vi "dragNode.vi"(8 "error in (no error)":errorcluster, 10 "Node Path":string, 11 "xceRootNode in":refnum<class "xceRootNode.lvclass">) -> (0 "error out":errorcluster, 3 "xceRootNode out":refnum<class "xceRootNode.lvclass">)   [LabVIEW 2013, in "xceRootNode.lvclass"]
doc: "Used in a drag/drop operation, when the user has detrmined which tree tag in a tree control they would like to drag."
uses:
  xceRootNode.lvclass
  xceDataNode/xceDataNode.lvclass
  xceRootNode.lvclass/xceRootNode.ctl
  xceNode/xceNode.lvclass
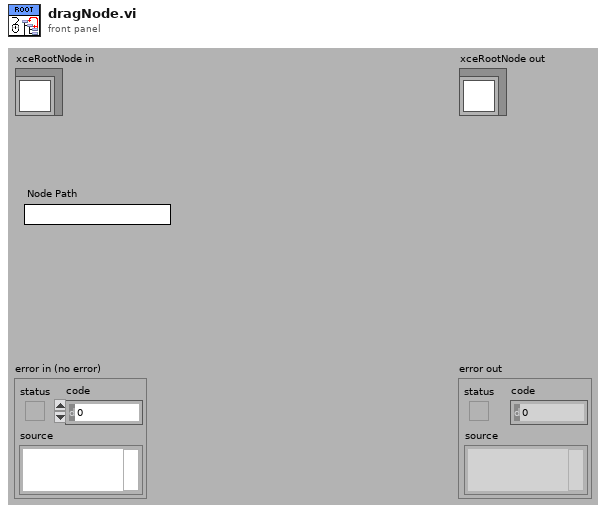
[diagram p1: front panel]
types:
  T1 = cluster{"data name":string, "drag data":variant}[]
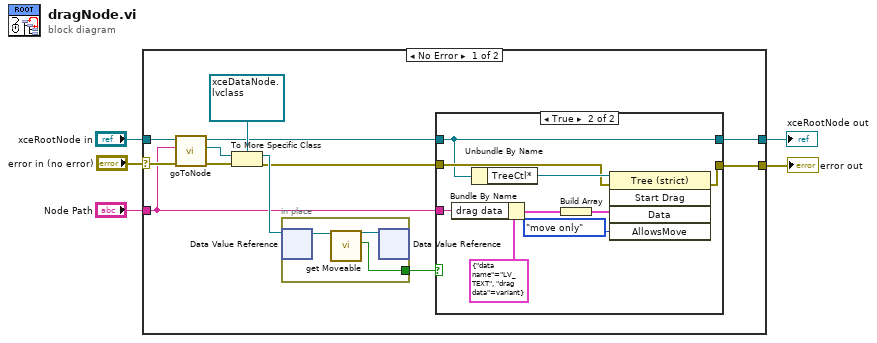
[diagram p0: block diagram]
diagram:
  n1 = case shown="No Error" "error in (no error)" {
    selector: "error in (no error)" -> [w14 w33]
    tunnel: [w8 w33] -> w4
    tunnel: [w6 w32] -> w2
    tunnel: "xceRootNode in" -> [w17 w32]
    tunnel: "Node Path" -> [w10 _]
    frame No Error {
      n2 = call "goToNode.vi"("error in (no error)"=w14, "Node Path"=w10, "xceNode in"=w17) -> ("error out"=w15:errorcluster, "goToNode* out"=w16:refnum<data-value>, "xceNode out"=w11:refnum<class "xceRootNode.lvclass">)  [unwired: 6 in]
      n3 = To More Specific Class(target class=refnum<data-value> refnum ("data value reference"), reference=w16, error in=w15) -> (specific class reference=w12:refnum<data-value>, error out=w9:errorcluster)
      n4 = in-place {
        in-place-border: [w29] -> w7
        n5 = in-place-dvr #1(w12) -> (w31:refnum<class "xceDataNode.lvclass">)  [unwired: 1 out]
        n6 = call "get Moveable.vi"("xceDataNode in"=w31) -> ("Moveable"=w29:bool, "xceDataNode out"=w30:refnum<class "xceDataNode.lvclass">)  [unwired: 8 in, 1 out]
        n7 = in-place-dvr #1(w30) -> ()  [unwired: 2 out]
      }
      n8 = case shown="True" w7 {
        tunnel: w11 -> [w19 w20]
        tunnel: w10 -> [_ w24]
        tunnel: w9 -> [w18 w22]
        tunnel: [w18 w21] -> w8
        tunnel: [w19 w20] -> w6
        frame False {
        }
        frame True {
          n9 = Bundle By Name(cluster=cluster{"data name":string, "drag data":variant} {"data name"="LV_TEXT", "drag data"=variant}, "drag data"=w24) -> (w23:cluster{"data name":string, "drag data":variant})
          n10 = Unbundle By Name(w20) -> ("TreeCtl*"=w28:refnum<vi>)
          n11 = Build Array(w23) -> (w26:T1)
          n12 = invoke class="Tree (strict)" method="Start Drag"(reference=w28, error in=w22, "Data"=w26, "AllowsMove"=enum32{"copy or move", "copy only", "move only"}."move only" ("Drag Mode")) -> (error out=w21:errorcluster)  [unwired: 1 in, 4 out]
        }
      }
    }
    frame Error {
    }
  }
  "error out" <- w4
  "xceRootNode out" <- w2
